vi "GetServoState.vi"(0 "Handle":u32, 1 "Controller Channel":i32) -> (7 "FT_Status":u32(ring) items=["FT_OK", "FT_INVALID_HANDLE", "FT_DEVICE_NOT_FOUND", "FT_DEVICE_NOT_OPENED", "FT_IO_ERROR", "FT_INSUFFICIENT_RESOURCES", "FT_INVALID_PARAMETER", "FT_INVALID_BAUD_RATE", "FT_DEVICE_NOT_OPENED_FOR_ERASE", "FT_DEVICE_NOT_OPENED_FOR_WRITE", "FT_FAILED_TO_WRITE_DEVICE", "FT_EEPROM_READ_FAILED", "FT_EEPROM_WRITE_FAILED", "FT_EEPROM_ERASE_FAILED", "FT_EEPROM_NOT_PRESENT", "FT_EEPROM_NOT_PROGRAMMED", "FT_INVALID_ARGS", "FT_NOT_SUPPORTED", "FT_OTHER_ERROR"], 9 "Servo State":i32)   [LabVIEW 2011]
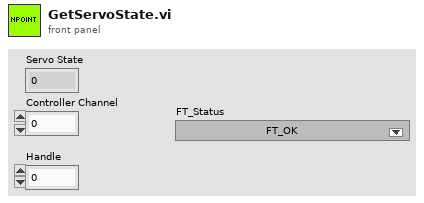
[diagram p1: front panel]
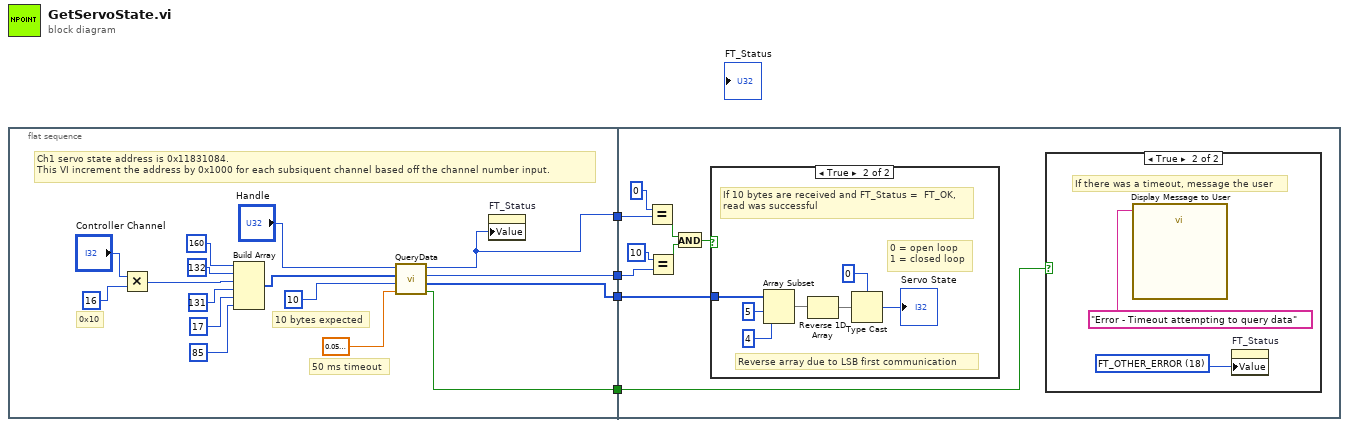
[diagram p0: block diagram]
diagram:
  n1 = flat-sequence {
    tunnel: [w9] -> w4
    tunnel: [w8] -> w3
    tunnel: [w7] -> w2
    tunnel: [w6] -> w1
    tunnel: w4 -> [w29]
    tunnel: w3 -> [w27]
    tunnel: w2 -> [w26]
    tunnel: w1 -> [w24]
    frame #0 {
      # "10 bytes expected"
      # "50 ms timeout"
      # "Ch1 servo state address is 0x11831084.\nThis VI increment the address by 0x1000 for each subsiquent channel based off the channel number input."
      # "0x10"
      n2 = Multiply(x="Controller Channel", y=u8 16) -> (x*y=w5:i32)
      n3 = Build Array(u8 160 ("element"), u8 132 ("element"), w5, u8 131 ("element"), u8 17 ("element"), u8 85 ("element")) -> (w12:i32[])
      n4 = call "QueryData.vi"("TimeoutLengthSeconds"=sgl 0.05, "NumBytesExpected"=u32 10, "Message"=w12, "Handle"="Handle") -> ("Timeout"=w7:bool, "Return Array"=w8:u8[], "Bytes Read"=w9:u32, "FT_Status"=w6:u32)  [unwired: 4 in]
      n5 = property on="FT_Status" class="Ring (strict)"("Value"=w6) -> ()  [unwired: 2 in, 2 out]
    }
    frame #1 {
      n6 = Equal?(x=u32 0, y=w24) -> (x = y?=w22:bool)
      n7 = Equal?(x=u32 10, y=w29) -> (x = y?=w23:bool)
      n8 = And(x=w22, y=w23) -> (x .and. y?=w21:bool)
      n9 = case shown="True" w21 {
        tunnel: w27 -> [_ w38]
        frame False {
        }
        frame True {
          # "0 = open loop\n1 = closed loop"
          # "Reverse array due to LSB first communication"
          # "If 10 bytes are received and FT_Status =  FT_OK,\nread was successful"
          n10 = Array Subset(array=w38, index=5, length=4) -> (w34:u8[])
          n11 = Reverse 1D Array(array=w34) -> (reversed array=w33:u8[])
          n12 = Type Cast(type=0, x=w33) -> (*(type *) &x=→"Servo State":i32)
        }
      }
      n13 = case shown="True" w26 {
        frame False {
        }
        frame True {
          w30 = u32 18 items=["FT_OK", "FT_INVALID_HANDLE", "FT_DEVICE_NOT_FOUND", "FT_DEVICE_NOT_OPENED", "FT_IO_ERROR", "FT_INSUFFICIENT_RESOURCES", "FT_INVALID_PARAMETER", "FT_INVALID_BAUD_RATE", "FT_DEVICE_NOT_OPENED_FOR_ERASE", "FT_DEVICE_NOT_OPENED_FOR_WRITE", "FT_FAILED_TO_WRITE_DEVICE", "FT_EEPROM_READ_FAILED", "FT_EEPROM_WRITE_FAILED", "FT_EEPROM_ERASE_FAILED", "FT_EEPROM_NOT_PRESENT", "FT_EEPROM_NOT_PROGRAMMED", "FT_INVALID_ARGS", "FT_NOT_SUPPORTED", "FT_OTHER_ERROR"] ("FT_Status")
          # "If there was a timeout, message the user"
          n14 = call "Display Message to User"("Message"="Error - Timeout attempting to query data") -> ()  [unwired: 9 in, 2 out]
          n15 = property on="FT_Status" class="Ring (strict)"("Value"=w30) -> ()  [unwired: 2 in, 2 out]
        }
      }
    }
  }
